vi "Wave-Find Chunk.vi"(8 "error in (no error)":errorcluster, 10 "Chunk ID":string, 11 "Refnum":refnum<file>) -> (0 "error out":errorcluster, 2 "chunk info":T1, 3 "refnum out":refnum<file>)   [LabVIEW 2020]
uses:
  Wave-Chunk Info.ctl
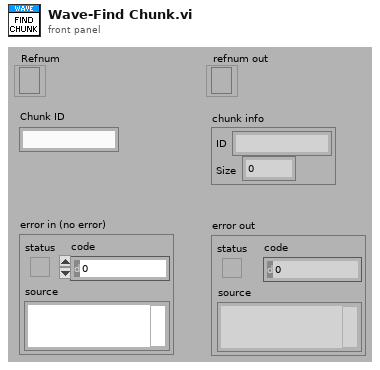
[diagram p1: front panel]
types:
  T1 = typedef "Wave-Chunk Info.ctl" = cluster{"ID":string, "Size":u32}
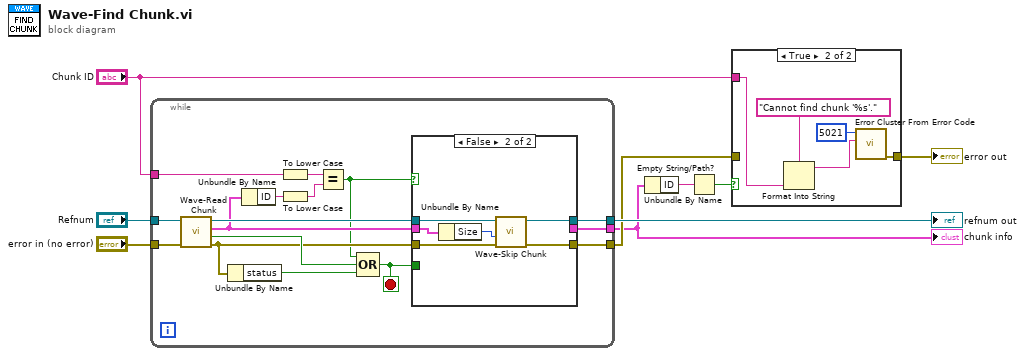
[diagram p0: block diagram]
diagram:
  n1 = while {
    tunnel: "Refnum" -> [w25]
    tunnel: [w20] -> w7
    tunnel: "error in (no error)" -> [w24]
    tunnel: [w18] -> w4
    tunnel: "Chunk ID" -> [w15]
    tunnel: [w12] -> w3
    stop <- w13 stop-if-true
    n2 = call "Wave-Read Chunk.vi"("error in (no error)"=w24, "refnum"=w25) -> ("error out"=w19:errorcluster, "EOF?"=w22:bool, "chunk info"=w17:T1, "refnum out"=w21:refnum<file>)  [unwired: 6 in]
    n3 = Unbundle By Name(w19) -> ("status"=w23:bool)
    n4 = Unbundle By Name(w17) -> ("ID"=w11:string)
    n5 = To Lower Case(string=w15) -> (all lower case string=w14:string)
    n6 = To Lower Case(string=w11) -> (all lower case string=w16:string)
    n7 = Equal?(x=w14, y=w16) -> (x = y?=w10:bool)
    n8 = Compound Arithmetic op=OR(w10, w22, w23) -> (w13:bool)
    n9 = case shown="False" w10 {
      tunnel: w21 -> [w28 w34]
      tunnel: [w26 w31] -> w18
      tunnel: w19 -> [w26 w32]
      tunnel: w17 -> [w27 w30]
      tunnel: [w28 w33] -> w20
      tunnel: w13 -> [_ _]
      tunnel: [w27 _] -> w12
      frame True {
      }
      frame False, Default {
        n10 = Unbundle By Name(w30) -> ("Size"=w29:u32)
        n11 = call "Wave-Skip Chunk.vi"("error in (no error)"=w32, "Total bytes"=w29, "refnum"=w34) -> ("error out"=w31:errorcluster, "refnum out"=w33:refnum<file>)  [unwired: 7 in]
      }
    }
  }
  "refnum out" <- w7
  "chunk info" <- w3
  n12 = Unbundle By Name(w3) -> ("ID"=w6:string)
  n13 = Empty String/Path?(string/path=w6) -> (empty?=w5:bool)
  n14 = case shown="True" w5 {
    tunnel: w4 -> [w35 _]
    tunnel: [w35 w40] -> w2
    tunnel: "Chunk ID" -> [_ w36]
    frame False {
    }
    frame True {
      n15 = Format Into String(format string="Cannot find chunk '%s'.", w36) -> (resulting string=w38:string)  [unwired: 2 in, 1 out]
      n16 = call <vilib>:"Error Cluster From Error Code.vi"("error message (\"\")"=w38, "error code (0)"=5021) -> ("error out"=w40:errorcluster)  [unwired: 7 in]
    }
  }
  "error out" <- w2
